vi "MIF-N_num_discr-de-obs.vi"(9 "X-NUM-D":dbl[](array[numeric]), 11 "X-NUM-MIF":dbl[](array[numeric])) -> (2 "N-NUM-MIF":i32[](array[numeric]))   [LabVIEW 2010, in "lv_02.lvlib"]
doc: "On compte le nombre d'occurrences de X-NUM-Discrète (valeurs observées) à partir de X-NUM-discrete-MIF (valeurs possibles)"
uses:
  lv_02.lvlib
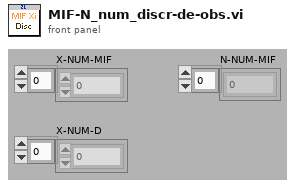
[diagram p1: front panel]
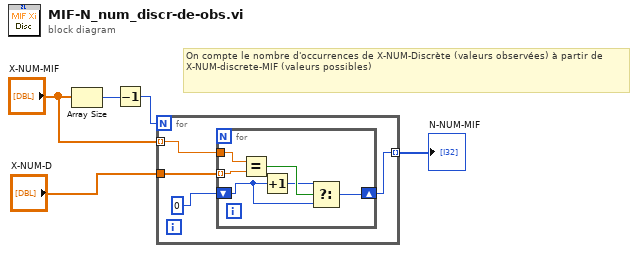
[diagram p0: block diagram]
diagram:
  # "On compte le nombre d'occurrences de X-NUM-Discrète (valeurs observées) à partir de X-NUM-discrete-MIF (valeurs possibles)"
  n1 = Array Size(array="X-NUM-MIF") -> (size(s)=w4:i32)
  n2 = Decrement(x=w4) -> (x-1=w5:i32)
  n3 = for {
    N: w5 -> [_]
    tunnel: "X-NUM-D" -> [w9]
    tunnel: "X-NUM-MIF" -> [w8] mode=indexing
    tunnel: [w6] -> w1 mode=indexing
    n4 = for {
      tunnel: w9 -> [w10] mode=indexing
      tunnel: w8 -> [w11]
      shift-right: [w15] -> w6
      shift-left: 0 -> [w12]
      n5 = Equal?(x=w11, y=w10) -> (x = y?=w14:bool)
      n6 = Increment(x=w12) -> (x+1=w13:i32)
      n7 = Select(t=w13, s=w14, f=w12) -> (s? t:f=w15:i32)
    }
  }
  "N-NUM-MIF" <- w1
